vi "NewP_req.vi"(6 "Static values":T1, 7 "Requeriments_boolean":T4, 8 "error in (no error)":errorcluster, 10 "Data Model in":T2, 11 "Reqs_cluster":T5) -> (0 "error out":errorcluster, 2 "Data Model out":T2)   [LabVIEW 2017]
uses:
  CONTROLS/Reqs_cluster.ctl
  CONTROLS/Requirements_boolean.ctl
  CONTROLS/Datamodel_FULL.ctl
  CONTROLS/P_ch_vs_SOC (array).ctl
  CONTROLS/Static_values.ctl
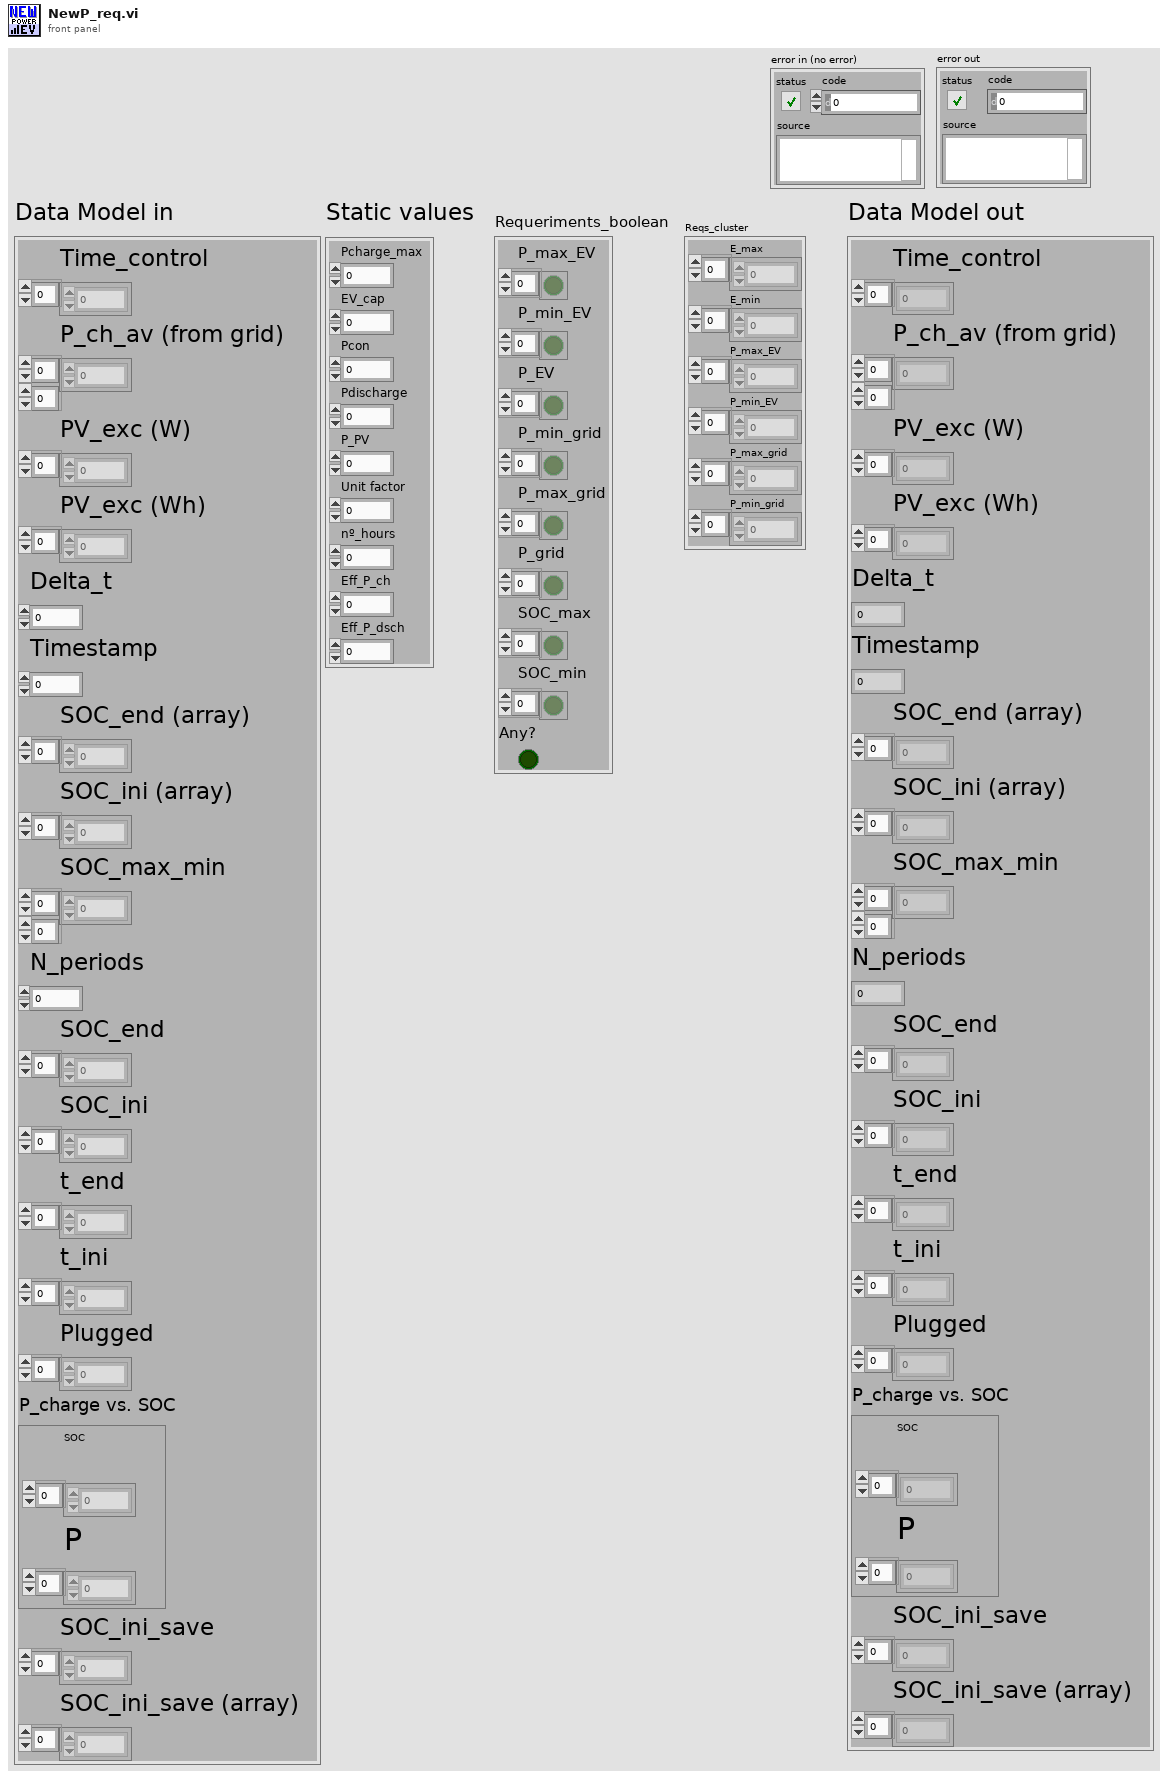
[diagram p1: front panel]
types:
  T1 = typedef "Static_values.ctl" = cluster{"Pcharge_max":dbl, "EV_cap":dbl, "Pcon":dbl, "Pdischarge":dbl, "P_PV":dbl, "Unit factor":dbl, "nº_hours":dbl, "Eff_P_ch":dbl, "Eff_P_dsch":dbl}
  T2 = typedef "Datamodel_FULL.ctl" = cluster{"Time_control":i32[], "P_ch_av (from grid)":dbl[][], "PV_exc (W)":dbl[], "PV_exc (Wh)":dbl[], "Delta_t":dbl, "Timestamp":i32, "SOC_end (array)":dbl[], "SOC_ini (array)":dbl[], "SOC_max_min":dbl[][], "N_periods":i32, "SOC_end":dbl[], "SOC_ini":dbl[], "t_end":i32[], "t_ini":i32[], "Plugged":i32[], "P_charge vs. SOC":T3, "SOC_ini_save":dbl[], "SOC_ini_save (array)":dbl[]}
  T3 = typedef "P_ch_vs_SOC (array).ctl" = cluster{"SOC":dbl[], "P":dbl[]}
  T4 = typedef "Requirements_boolean.ctl" = cluster{"P_max_EV":bool[], "P_min_EV":bool[], "P_EV":bool[], "P_min_grid":bool[], "P_max_grid":bool[], "P_grid":bool[], "SOC_max":bool[], "SOC_min":bool[], "Any?":bool}
  T5 = typedef "Reqs_cluster.ctl" = cluster{"E_max":dbl[], "E_min":dbl[], "P_max_EV":dbl[], "P_min_EV":dbl[], "P_max_grid":dbl[], "P_min_grid":dbl[]}
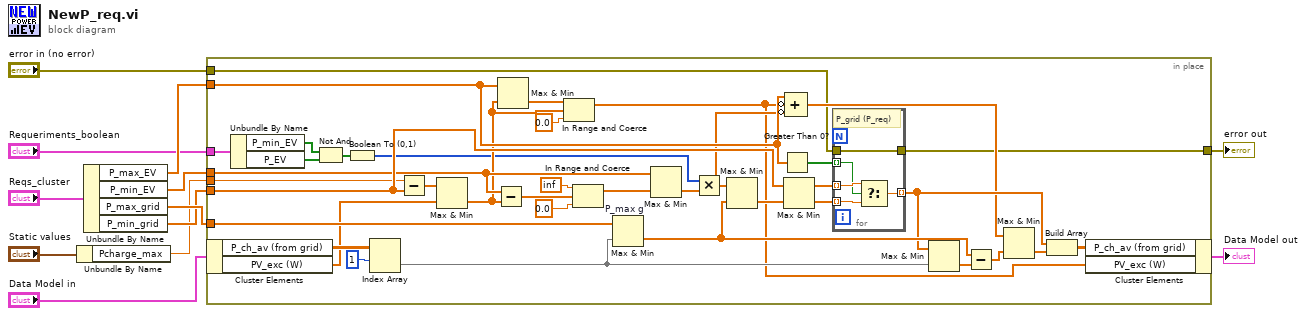
[diagram p0: block diagram]
diagram:
  n1 = Unbundle By Name("Static values") -> ("Pcharge_max"=w6:dbl)
  n2 = Unbundle By Name("Reqs_cluster") -> ("P_max_EV"=w9:dbl[], "P_min_EV"=w8:dbl[], "P_max_grid"=w11:dbl[], "P_min_grid"=w10:dbl[])
  n3 = in-place {
    in-place-border: w11 -> [w50]
    in-place-border: w10 -> [w49]
    in-place-border: w9 -> [w48]
    in-place-border: w8 -> [w47]
    in-place-border: w6 -> [w20]
    in-place-border: "error in (no error)" -> [w15]
    in-place-border: [w14] -> w2
    in-place-border: "Requeriments_boolean" -> [w13]
    n4 = in-place-cluster #1("Data Model in") -> ("P_ch_av (from grid)"=w17:dbl[][], "PV_exc (W)"=w16:dbl[])
    n5 = Unbundle By Name(w13) -> ("P_min_EV"=w42:bool[], "P_EV"=w43:bool[])
    n6 = Not And(1:w43, 2:w42) -> (0:w30:bool[])
    n7 = Boolean To (0,1)(Boolean=w30) -> (0, 1=w21:i16[])
    n8 = Index Array(array=w17, index (row)=1) -> (element=w38:dbl[])  [unwired: 1 in]
    n9 = Subtract(x=w20, y=w49) -> (x-y=w44:dbl[])
    n10 = Max & Min(x=w44, y=w16) -> (min(x,y)=w25:dbl[])  [unwired: 1 out]
    n11 = Subtract(x=w47, y=w25) -> (x-y=w35:dbl[])
    n12 = Max & Min(x=w48, y=w25) -> (min(x,y)=w24:dbl[])  [unwired: 1 out]
    n13 = In Range and Coerce(upper limit=w24, x=w25, lower limit=0.0 ("t")) -> (coerced(x)=w18:dbl[])  [unwired: 1 out]
    n14 = In Range and Coerce(upper limit=inf, x=w35, lower limit=0.0) -> (coerced(x)=w36:dbl[])  [unwired: 1 out]
    n15 = Max & Min "P_max g"(x=w50, y=w38) -> (min(x,y)=w45:dbl[])  [unwired: 1 out]
    n16 = Max & Min(x=w47, y=w36) -> (min(x,y)=w23:dbl[])  [unwired: 1 out]
    n17 = Multiply(x=w21, y=w23) -> (x*y=w31:dbl[])
    n18 = Max & Min(x=w31, y=w45) -> (min(x,y)=w26:dbl[])  [unwired: 1 out]
    n19 = Greater Than 0?(x=w48) -> (x > 0?=w29:bool[])
    n20 = Max & Min(x=w49, y=w26) -> (max(x,y)=w27:dbl[], min(x,y)=w28:dbl[])
    n21 = Compound Arithmetic op=ADD(w48, invert w18, invert w31) -> (w32:dbl[])
    n22 = for {
      tunnel: [w55] -> w40 mode=indexing
      tunnel: w27 -> [w54] mode=indexing
      tunnel: w28 -> [w53] mode=indexing
      tunnel: w29 -> [w52] mode=indexing
      tunnel: w15 -> [w51]
      tunnel: [w51] -> w14
      # "P_grid (P_req)"
      n23 = Select(t=w54, s=w52, f=w53) -> (s? t:f=w55:dbl)
    }
    n24 = Max & Min(x=w40, y=w38) -> (min(x,y)=w46:dbl[])  [unwired: 1 out]
    n25 = Subtract(x=w45, y=w46) -> (x-y=w37:dbl[])
    n26 = Max & Min(x=w32, y=w37) -> (min(x,y)=w41:dbl[])  [unwired: 1 out]
    n27 = Build Array(w40, w41) -> (w19:dbl[][])
    n28 = in-place-cluster #1("P_ch_av (from grid)"=w19, "PV_exc (W)"=w18) -> (→"Data Model out":T2)
  }
  "error out" <- w2
